vi "getParAndRowChkRes.vi"(4 "Row number":u32, 6 "arg":string, 7 "table":string[][](array[string]), 8 "error in":errorcluster, 9 "function":string, 10 "section":string, 11 "Tree Refnum in":refnum<vi>) -> (0 "error out":errorcluster, 1 "Check result":string="√", 2 "par":string, 3 "Tree Refnum out":refnum<vi>)   [LabVIEW 2010]
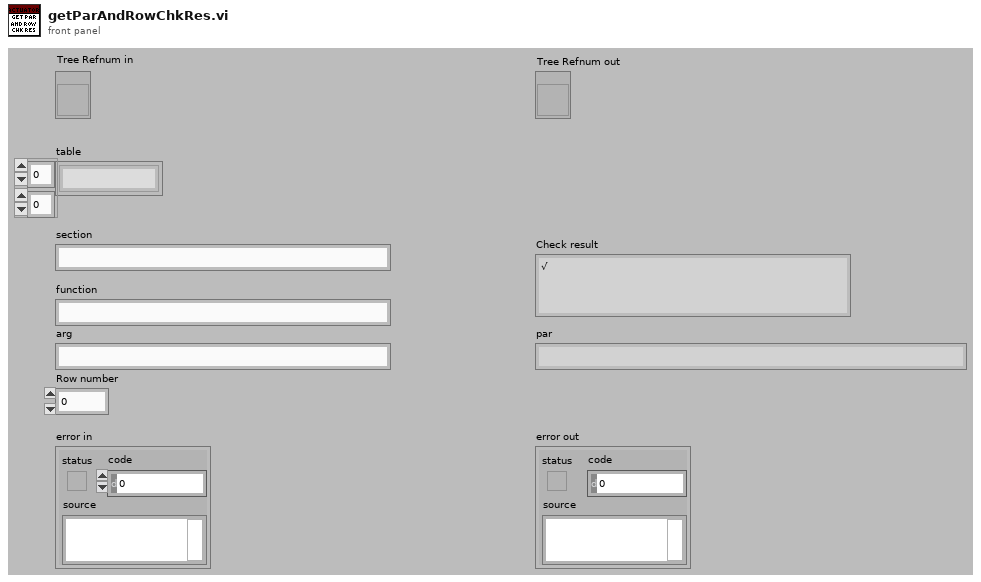
[diagram p1: front panel]
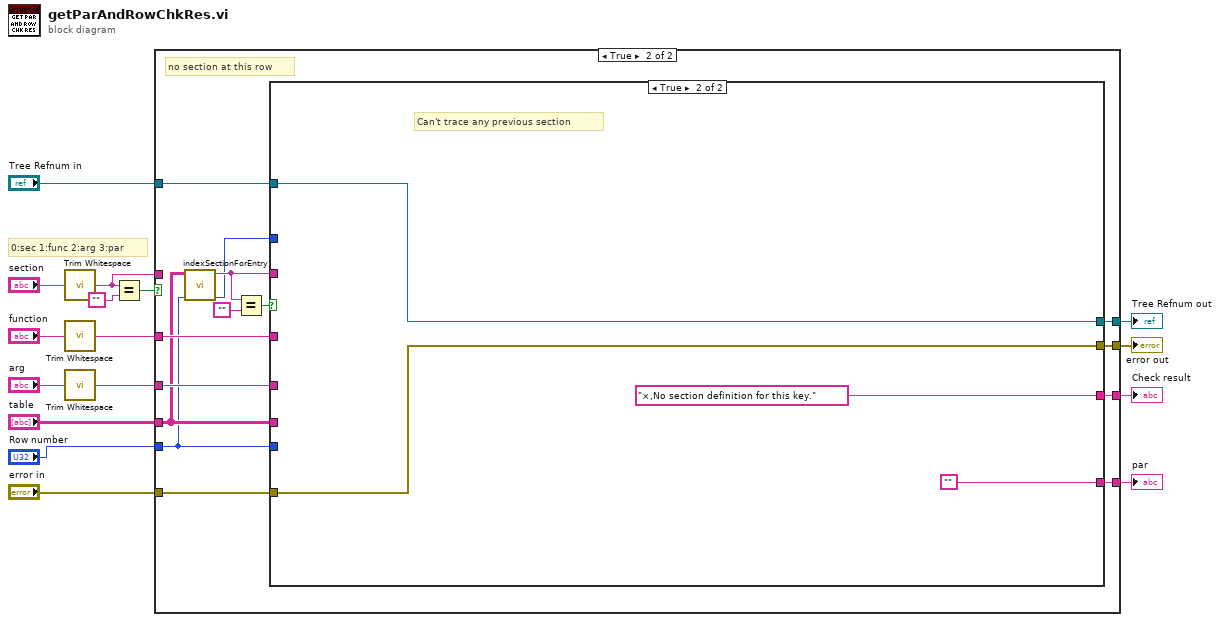
[diagram p0: block diagram]
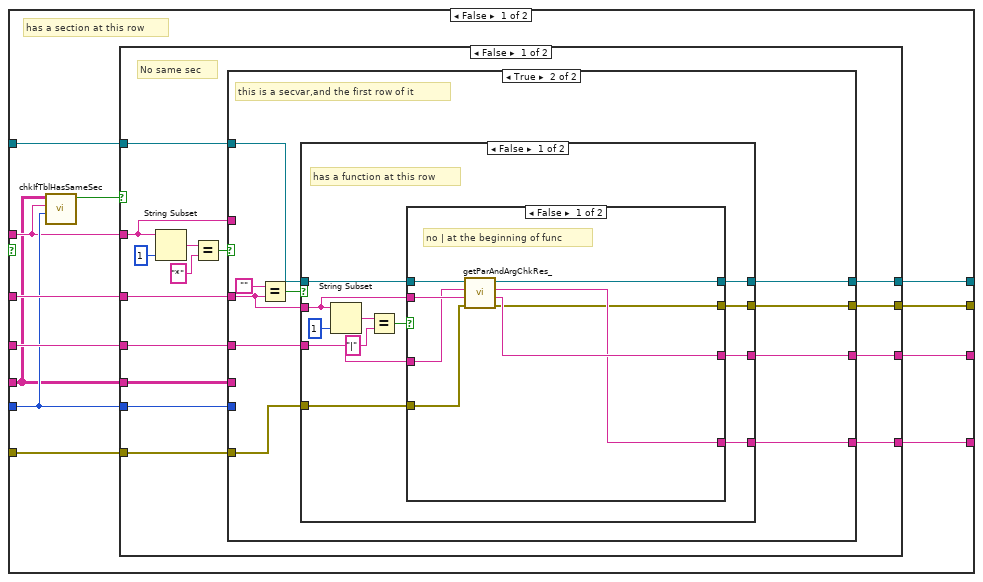
[diagram p2: hidden frame]
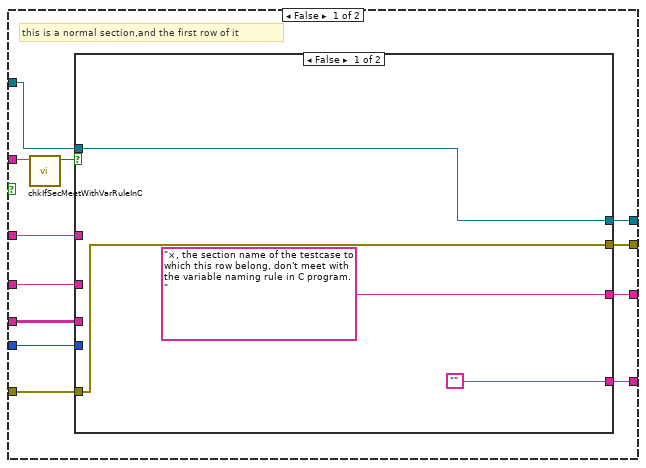
[diagram p3: hidden frame]
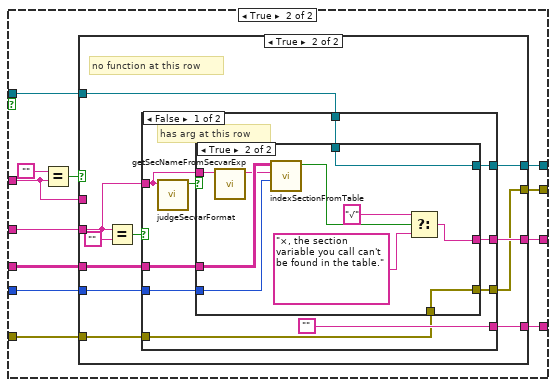
[diagram p4: hidden frame]
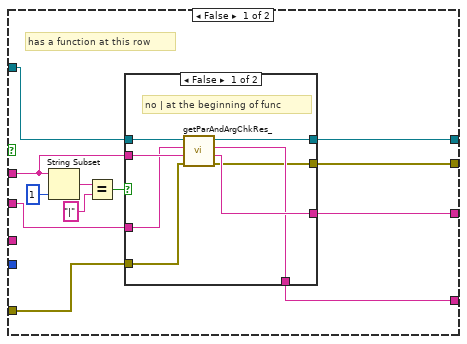
[diagram p5: hidden frame]
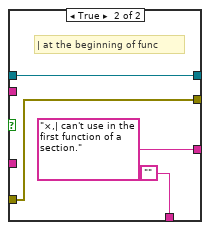
[diagram p6: hidden frame]
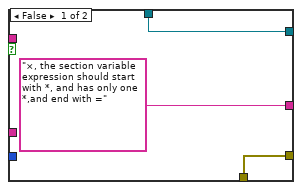
[diagram p7: hidden frame]
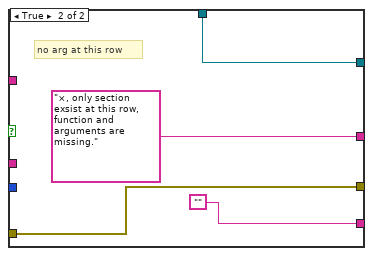
[diagram p8: hidden frame]
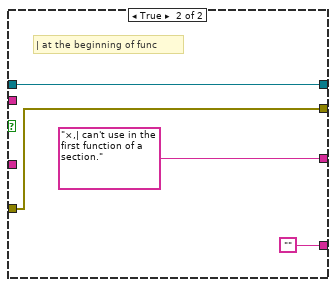
[diagram p9: hidden frame]
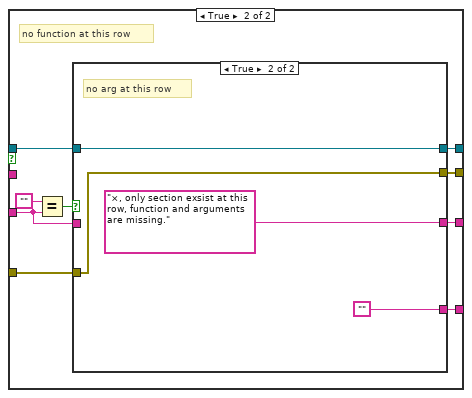
[diagram p10: hidden frame]
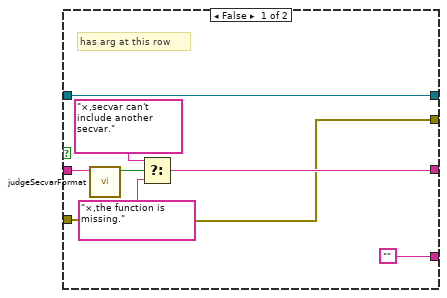
[diagram p11: hidden frame]
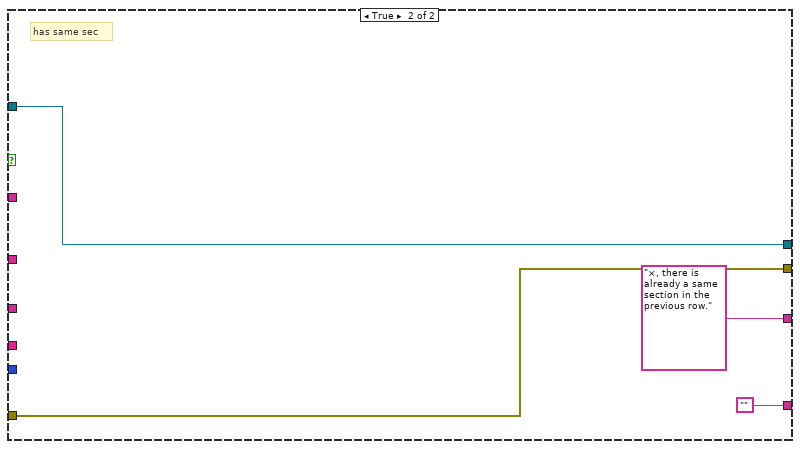
[diagram p12: hidden frame]
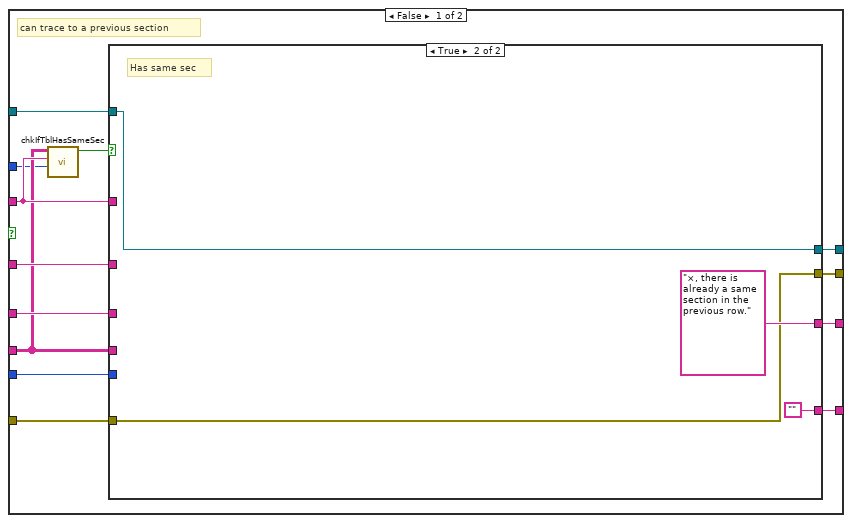
[diagram p13: hidden frame]
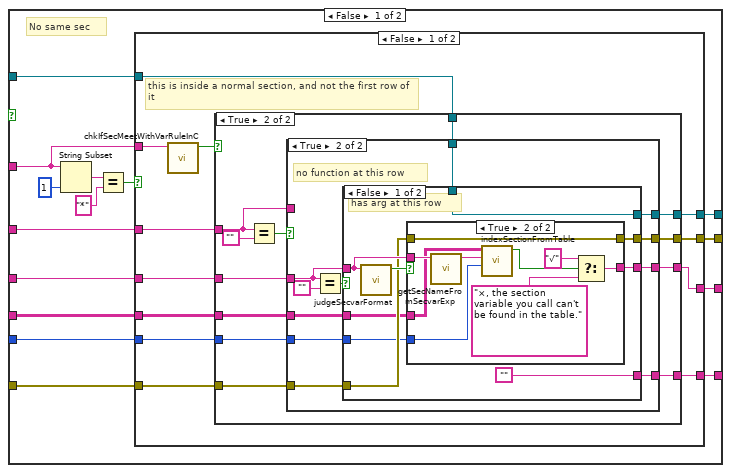
[diagram p14: hidden frame]
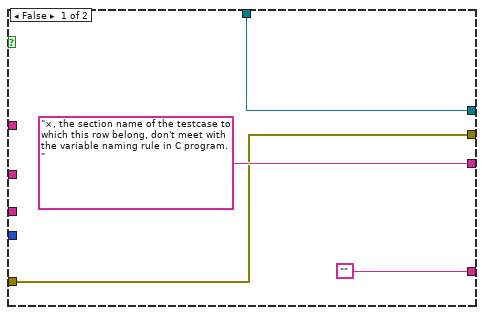
[diagram p15: hidden frame]
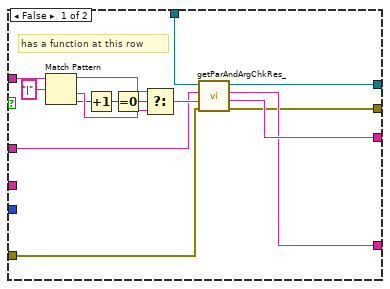
[diagram p16: hidden frame]
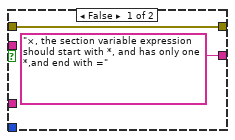
[diagram p17: hidden frame]
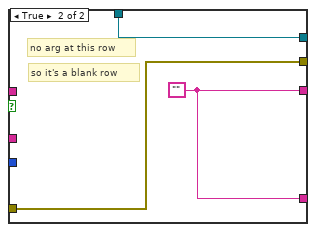
[diagram p18: hidden frame]
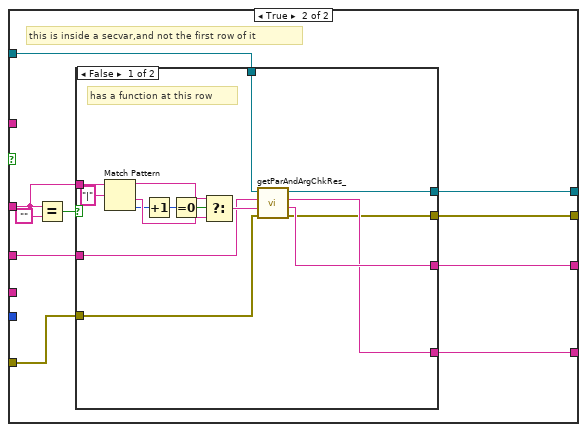
[diagram p19: hidden frame]
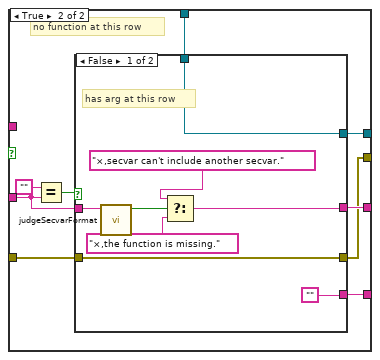
[diagram p20: hidden frame]
diagram:
  # "0:sec 1:func 2:arg 3:par"
  n1 = call <vilib>:"Trim Whitespace.vi"("string"="section") -> ("trimmed string"=w11:string)  [unwired: 1 in]
  n2 = call <vilib>:"Trim Whitespace.vi"("string"="function") -> ("trimmed string"=w14:string)  [unwired: 1 in]
  n3 = call <vilib>:"Trim Whitespace.vi"("string"="arg") -> ("trimmed string"=w13:string)  [unwired: 1 in]
  n4 = Equal?(x=w11, y="") -> (x = y?=w15:bool)
  n5 = case shown="True" w15 {
    tunnel: w14 -> [w28 w204]
    tunnel: w13 -> [w27 w203]
    tunnel: "Tree Refnum in" -> [w26 w202]
    tunnel: w11 -> [w19 _]
    tunnel: [w25 w201] -> w10
    tunnel: [w24 w200] -> w9
    tunnel: [w23 w199] -> w3
    tunnel: [w21 w198] -> w4
    tunnel: "error in" -> [w22 w197]
    tunnel: "table" -> [w18 w195]
    tunnel: "Row number" -> [w20 w194]
    frame False {
      # "has a section at this row"
      n6 = call "chkIfTblHasSameSec.vi"("rowNumAtWhichSecExist"=w20, "Section"=w19, "tbl"=w18) -> ("foundSameSec?"=w17:bool)  [unwired: 8 in]
      n7 = case shown="False" w17 {
        tunnel: w28 -> [w39 _]
        tunnel: w27 -> [w38 _]
        tunnel: w26 -> [w37 w190]
        tunnel: [w36 w190] -> w25
        tunnel: [w35 "×, there is already a same section in the previous row."] -> w24
        tunnel: [w34 ""] -> w23
        tunnel: w22 -> [w33 w189]
        tunnel: [w32 w189] -> w21
        tunnel: w20 -> [w31 _]
        tunnel: w19 -> [w30 _]
        tunnel: w18 -> [w29 _]
        frame False {
          # "No same sec"
          n8 = String Subset(string=w30, length (rest)=1 ("length (rest)")) -> (substring=w43:string)  [unwired: 1 in]
          n9 = Equal?(x=w43, y="*") -> (x = y?=w40:bool)
          n10 = case shown="True" w40 {
            tunnel: w39 -> [w53 w140]
            tunnel: w38 -> [w52 w141]
            tunnel: w37 -> [w51 w139]
            tunnel: w30 -> [w55 _]
            tunnel: [w50 w138] -> w36
            tunnel: [w49 w137] -> w35
            tunnel: [w48 w136] -> w34
            tunnel: w33 -> [w47 w135]
            tunnel: [w46 w134] -> w32
            tunnel: w29 -> [w45 _]
            tunnel: w31 -> [w44 _]
            frame False {
              # "this is a normal section,and the first row of it"
              n11 = call "chkIfSecMeetWithVarRuleInC.vi"("section"=w55) -> ("meetWithVarRuleInC?"=w54:bool)  [unwired: 10 in]
              n12 = case shown="False" w54 {
                tunnel: w53 -> [_ w68]
                tunnel: w52 -> [_ w69]
                tunnel: w51 -> [w59 w67]
                tunnel: [w59 w66] -> w50
                tunnel: ["×, the section name of the testcase to which this row belong, don't meet with the variable naming rule in C program." w65] -> w49
                tunnel: ["" w64] -> w48
                tunnel: w47 -> [w56 w62]
                tunnel: [w56 w63] -> w46
                tunnel: w45 -> [_ w61]
                tunnel: w44 -> [_ w60]
                frame False {
                }
                frame True {
                  n13 = Equal?(x="", y=w68) -> (x = y?=w70:bool)
                  n14 = case shown="True" w70 {
                    tunnel: w69 -> [w79 w104]
                    tunnel: w68 -> [w77 _]
                    tunnel: w67 -> [w78 w102]
                    tunnel: [w76 w103] -> w66
                    tunnel: [w75 w101] -> w65
                    tunnel: [w74 w100] -> w64
                    tunnel: [w73 w98] -> w63
                    tunnel: w62 -> [w72 w99]
                    tunnel: w61 -> [_ w97]
                    tunnel: w60 -> [_ w96]
                    frame False {
                      # "has a function at this row"
                      n15 = String Subset(string=w77, length (rest)=1 ("length (rest)")) -> (substring=w82:string)  [unwired: 1 in]
                      n16 = Equal?(x=w82, y="|" ("regular expression")) -> (x = y?=w81:bool)
                      n17 = case shown="False" w81 {
                        tunnel: w77 -> [w91 _]
                        tunnel: w79 -> [w90 _]
                        tunnel: w78 -> [w89 w95]
                        tunnel: [w88 w95] -> w76
                        tunnel: [w87 "×,| can't use in the first function of a section."] -> w75
                        tunnel: [w86 ""] -> w74
                        tunnel: [w85 w92] -> w73
                        tunnel: w72 -> [w84 w92]
                        frame False {
                          # "no | at the beginning of func"
                          n18 = call "getParAndArgChkRes_.vi"("error in"=w84, "func"=w91, "arg"=w90, "Tree Refnum in"=w89) -> ("error out"=w85:errorcluster, "Check result"=w87:string, "par"=w86:string, "Tree Refnum out"=w88:refnum<vi>)  [unwired: 4 in]
                        }
                        frame True {
                          # "| at the beginning of func"
                        }
                      }
                    }
                    frame True {
                      # "no function at this row"
                      n19 = Equal?(x=w104, y="") -> (x = y?=w105:bool)
                      n20 = case shown="False" w105 {
                        tunnel: w104 -> [w111 _]
                        tunnel: [w113 w133] -> w103
                        tunnel: w102 -> [w112 w133]
                        tunnel: [w114 "×, only section exsist at this row, function and arguments are missing." ("Value")] -> w101
                        tunnel: ["" ""] -> w100
                        tunnel: w99 -> [w107 w130]
                        tunnel: [w108 w130] -> w98
                        tunnel: w97 -> [w110 _]
                        tunnel: w96 -> [w109 _]
                        frame False {
                          # "has arg at this row"
                          n21 = call "judgeSecvarFormat.vi"("section variable"=w111) -> ("correct format?"=w115:bool)  [unwired: 10 in]
                          n22 = case shown="True" w115 {
                            tunnel: ["×, the section variable expression should start with *, and has only one *,and end with =" ("Value") w121] -> w114
                            tunnel: [w118 w129] -> w113
                            tunnel: w112 -> [w118 w129]
                            tunnel: w111 -> [_ w128]
                            tunnel: w110 -> [_ w127]
                            tunnel: w109 -> [_ w125]
                            tunnel: [w117 w120] -> w108
                            tunnel: w107 -> [w117 w120]
                            frame False {
                            }
                            frame True {
                              n23 = call "getSecNameFromSecvarExp.vi"("secvarExp"=w128) -> ("secWith*"=w126:string)  [unwired: 10 in]
                              n24 = call "indexSectionFromTable.vi"("rowNum"=w125, "indexSec"=w126, "tbl"=w127) -> ("found?"=w124:bool)  [unwired: 8 in]
                              n25 = Select(t="√", s=w124, f="×, the section variable you call can't be found in the table." ("Value")) -> (s? t:f=w121:string)
                            }
                          }
                        }
                        frame True {
                          # "no arg at this row"
                        }
                      }
                    }
                  }
                }
              }
            }
            frame True {
              # "this is a secvar,and the first row of it"
              n26 = Equal?(x="", y=w140) -> (x = y?=w142:bool)
              n27 = case shown="False" w142 {
                tunnel: w141 -> [w150 w174]
                tunnel: w140 -> [w151 _]
                tunnel: w139 -> [w149 w172]
                tunnel: [w148 w173] -> w138
                tunnel: [w147 w171] -> w137
                tunnel: [w146 w170] -> w136
                tunnel: w135 -> [w145 w169]
                tunnel: [w144 w168] -> w134
                frame False {
                  # "has a function at this row"
                  n28 = String Subset(string=w151, length (rest)=1 ("length (rest)")) -> (substring=w153:string)  [unwired: 1 in]
                  n29 = Equal?(x=w153, y="|" ("regular expression")) -> (x = y?=w152:bool)
                  n30 = case shown="False" w152 {
                    tunnel: w151 -> [w163 _]
                    tunnel: w150 -> [w162 _]
                    tunnel: w149 -> [w161 w167]
                    tunnel: [w160 w167] -> w148
                    tunnel: [w159 "×,| can't use in the first function of a section."] -> w147
                    tunnel: [w158 ""] -> w146
                    tunnel: w145 -> [w157 w164]
                    tunnel: [w156 w164] -> w144
                    frame False {
                      # "no | at the beginning of func"
                      n31 = call "getParAndArgChkRes_.vi"("error in"=w157, "func"=w163, "arg"=w162, "Tree Refnum in"=w161) -> ("error out"=w156:errorcluster, "Check result"=w159:string, "par"=w158:string, "Tree Refnum out"=w160:refnum<vi>)  [unwired: 4 in]
                    }
                    frame True {
                      # "| at the beginning of func"
                    }
                  }
                }
                frame True {
                  # "no function at this row"
                  n32 = Equal?(x="", y=w174) -> (x = y?=w175:bool)
                  n33 = case shown="True" w175 {
                    tunnel: w174 -> [w184 _]
                    tunnel: [w180 w188] -> w173
                    tunnel: w172 -> [w180 w188]
                    tunnel: [w179 "×, only section exsist at this row, function and arguments are missing." ("Value")] -> w171
                    tunnel: ["" ""] -> w170
                    tunnel: w169 -> [w177 w185]
                    tunnel: [w177 w185] -> w168
                    frame False {
                      # "has arg at this row"
                      n34 = call "judgeSecvarFormat.vi"("section variable"=w184) -> ("correct format?"=w183:bool)  [unwired: 10 in]
                      n35 = Select(t="×,secvar can't include another secvar.", s=w183, f="×,the function is missing.") -> (s? t:f=w179:string)
                    }
                    frame True {
                      # "no arg at this row"
                    }
                  }
                }
              }
            }
          }
        }
        frame True {
          # "has same sec"
        }
      }
    }
    frame True {
      # "no section at this row"
      n36 = call "indexSectionForEntry.vi"("rowNum"=w194, "tbl"=w195) -> ("rowNumAtWhichSecExist"=w193:i32, "indexSection"=w196:string)  [unwired: 8 in]
      n37 = Equal?(x=w196, y="") -> (x = y?=w205:bool)
      n38 = case shown="True" w205 {
        tunnel: w196 -> [w210 _]
        tunnel: w204 -> [w219 _]
        tunnel: w203 -> [w218 _]
        tunnel: w202 -> [w217 w365]
        tunnel: [w216 w365] -> w201
        tunnel: [w215 "×,No section definition for this key."] -> w200
        tunnel: [w214 ""] -> w199
        tunnel: [w213 w362] -> w198
        tunnel: w197 -> [w212 w362]
        tunnel: w195 -> [w209 _]
        tunnel: w194 -> [w211 _]
        tunnel: w193 -> [w208 _]
        frame False {
          # "can trace to a previous section"
          n39 = call "chkIfTblHasSameSec.vi"("rowNumAtWhichSecExist"=w208, "Section"=w210, "tbl"=w209) -> ("foundSameSec?"=w207:bool)  [unwired: 8 in]
          n40 = case shown="True" w207 {
            tunnel: w219 -> [w230 _]
            tunnel: w218 -> [w229 _]
            tunnel: w217 -> [w228 w361]
            tunnel: [w227 w361] -> w216
            tunnel: [w226 "×, there is already a same section in the previous row."] -> w215
            tunnel: [w225 ""] -> w214
            tunnel: [w224 w359] -> w213
            tunnel: w212 -> [w223 w359]
            tunnel: w211 -> [w222 _]
            tunnel: w210 -> [w221 _]
            tunnel: w209 -> [w220 _]
            frame False {
              # "No same sec"
              n41 = String Subset(string=w221, length (rest)=1 ("length (rest)")) -> (substring=w233:string)  [unwired: 1 in]
              n42 = Equal?(x=w233, y="*") -> (x = y?=w231:bool)
              n43 = case shown="False" w231 {
                tunnel: w230 -> [w244 w318]
                tunnel: w229 -> [w243 w319]
                tunnel: w228 -> [w242 w317]
                tunnel: w221 -> [w246 _]
                tunnel: [w241 w316] -> w227
                tunnel: [w240 w315] -> w226
                tunnel: [w239 w314] -> w225
                tunnel: [w238 w313] -> w224
                tunnel: w223 -> [w237 w312]
                tunnel: w220 -> [w236 _]
                tunnel: w222 -> [w235 _]
                frame False {
                  # "this is inside a normal section, and not the first row of it"
                  n44 = call "chkIfSecMeetWithVarRuleInC.vi"("section"=w246) -> ("meetWithVarRuleInC?"=w245:bool)  [unwired: 10 in]
                  n45 = case shown="True" w245 {
                    tunnel: w244 -> [_ w259]
                    tunnel: w243 -> [_ w260]
                    tunnel: w242 -> [w250 w258]
                    tunnel: [w250 w257] -> w241
                    tunnel: ["×, the section name of the testcase to which this row belong, don't meet with the variable naming rule in C program." w256] -> w240
                    tunnel: ["" w255] -> w239
                    tunnel: [w247 w254] -> w238
                    tunnel: w237 -> [w247 w253]
                    tunnel: w236 -> [_ w252]
                    tunnel: w235 -> [_ w251]
                    frame False {
                    }
                    frame True {
                      n46 = Equal?(x=w259, y="") -> (x = y?=w261:bool)
                      n47 = case shown="True" w261 {
                        tunnel: w260 -> [w268 w286]
                        tunnel: w259 -> [w270 _]
                        tunnel: w258 -> [w269 w284]
                        tunnel: [w267 w285] -> w257
                        tunnel: [w266 w283] -> w256
                        tunnel: [w265 w282] -> w255
                        tunnel: [w264 w280] -> w254
                        tunnel: w253 -> [w263 w281]
                        tunnel: w252 -> [_ w279]
                        tunnel: w251 -> [_ w278]
                        frame False {
                          # "has a function at this row"
                          n48 = Match Pattern(string=w270, regular expression="|") -> (before substring=w276:string, after substring=w277:string, offset past match=w273:i32)  [unwired: 1 in, 1 out]
                          n49 = Increment(x=w273) -> (x+1=w274:i32)
                          n50 = Equal To 0?(x=w274) -> (x = 0?=w275:bool)
                          n51 = Select(t=w276, s=w275, f=w277) -> (s? t:f=w271:string)
                          n52 = call "getParAndArgChkRes_.vi"("error in"=w263, "func"=w271, "arg"=w268, "Tree Refnum in"=w269) -> ("error out"=w264:errorcluster, "Check result"=w266:string, "par"=w265:string, "Tree Refnum out"=w267:refnum<vi>)  [unwired: 4 in]
                        }
                        frame True {
                          # "no function at this row"
                          n53 = Equal?(x=w286, y="") -> (x = y?=w287:bool)
                          n54 = case shown="False" w287 {
                            tunnel: w286 -> [w293 _]
                            tunnel: [w297 w311] -> w285
                            tunnel: w284 -> [w297 w311]
                            tunnel: [w294 w310] -> w283
                            tunnel: ["" w310] -> w282
                            tunnel: w281 -> [w291 w309]
                            tunnel: [w292 w309] -> w280
                            tunnel: w279 -> [w290 _]
                            tunnel: w278 -> [w289 _]
                            frame False {
                              # "has arg at this row"
                              n55 = call "judgeSecvarFormat.vi"("section variable"=w293) -> ("correct format?"=w295:bool)  [unwired: 10 in]
                              n56 = case shown="True" w295 {
                                tunnel: ["×, the section variable expression should start with *, and has only one *,and end with =" ("Value") w304] -> w294
                                tunnel: w293 -> [_ w308]
                                tunnel: [w298 w303] -> w292
                                tunnel: w291 -> [w298 w303]
                                tunnel: w290 -> [_ w302]
                                tunnel: w289 -> [_ w301]
                                frame False {
                                }
                                frame True {
                                n57 = call "getSecNameFromSecvarExp.vi"("secvarExp"=w308) -> ("secWith*"=w307:string)  [unwired: 10 in]
                                n58 = call "indexSectionFromTable.vi"("rowNum"=w301, "indexSec"=w307, "tbl"=w302) -> ("found?"=w306:bool)  [unwired: 8 in]
                                n59 = Select(t="√", s=w306, f="×, the section variable you call can't be found in the table." ("Value")) -> (s? t:f=w304:string)
                                }
                              }
                            }
                            frame True {
                              w310 = ""
                              # "so it's a blank row"
                              # "no arg at this row"
                            }
                          }
                        }
                      }
                    }
                  }
                }
                frame True {
                  # "this is inside a secvar,and not the first row of it"
                  n60 = Equal?(x=w318, y="") -> (x = y?=w320:bool)
                  n61 = case shown="False" w320 {
                    tunnel: w319 -> [w327 w343]
                    tunnel: w318 -> [w330 _]
                    tunnel: w317 -> [w328 w341]
                    tunnel: [w326 w342] -> w316
                    tunnel: [w325 w340] -> w315
                    tunnel: [w324 w339] -> w314
                    tunnel: [w323 w337] -> w313
                    tunnel: w312 -> [w322 w338]
                    frame False {
                      # "has a function at this row"
                      n62 = Match Pattern(string=w330, regular expression="|") -> (before substring=w335:string, after substring=w336:string, offset past match=w332:i32)  [unwired: 1 in, 1 out]
                      n63 = Increment(x=w332) -> (x+1=w333:i32)
                      n64 = Equal To 0?(x=w333) -> (x = 0?=w334:bool)
                      n65 = Select(t=w335, s=w334, f=w336) -> (s? t:f=w329:string)
                      n66 = call "getParAndArgChkRes_.vi"("error in"=w322, "func"=w329, "arg"=w327, "Tree Refnum in"=w328) -> ("error out"=w323:errorcluster, "Check result"=w325:string, "par"=w324:string, "Tree Refnum out"=w326:refnum<vi>)  [unwired: 4 in]
                    }
                    frame True {
                      # "no function at this row"
                      n67 = Equal?(x="", y=w343) -> (x = y?=w344:bool)
                      n68 = case shown="False" w344 {
                        tunnel: w343 -> [w353 _]
                        tunnel: [w349 w357] -> w342
                        tunnel: w341 -> [w349 w357]
                        tunnel: [w348 ""] -> w340
                        tunnel: ["" ""] -> w339
                        tunnel: w338 -> [w346 w354]
                        tunnel: [w346 w354] -> w337
                        frame False {
                          # "has arg at this row"
                          n69 = call "judgeSecvarFormat.vi"("section variable"=w353) -> ("correct format?"=w352:bool)  [unwired: 10 in]
                          n70 = Select(t="×,secvar can't include another secvar.", s=w352, f="×,the function is missing.") -> (s? t:f=w348:string)
                        }
                        frame True {
                          # "so it's a blank row"
                          # "no arg at this row"
                        }
                      }
                    }
                  }
                }
              }
            }
            frame True {
              # "Has same sec"
            }
          }
        }
        frame True {
          # "Can't trace any previous section"
        }
      }
    }
  }
  "Check result" <- w9
  "error out" <- w4
  "Tree Refnum out" <- w10
  "par" <- w3
